vi "saveTestParameters.vi"(8 "error in (no error)":errorcluster, 11 "Logger in":refnum<class "TestDataLog.lvclass">) -> (0 "error out":errorcluster, 3 "Logger out":refnum<class "TestDataLog.lvclass">)   [LabVIEW 2013, in "TestDataLog.lvclass"]
uses:
  TestDataLog.lvclass
  <userlib>/Common/Log/Log/Log.lvclass/Log.ctl
  TestDataLog.lvclass/TestDataLog.ctl
  <vilib>/Utility/file.llb/Write To Spreadsheet File (string).vi
  <userlib>/Common/Log/Log/Log.lvclass
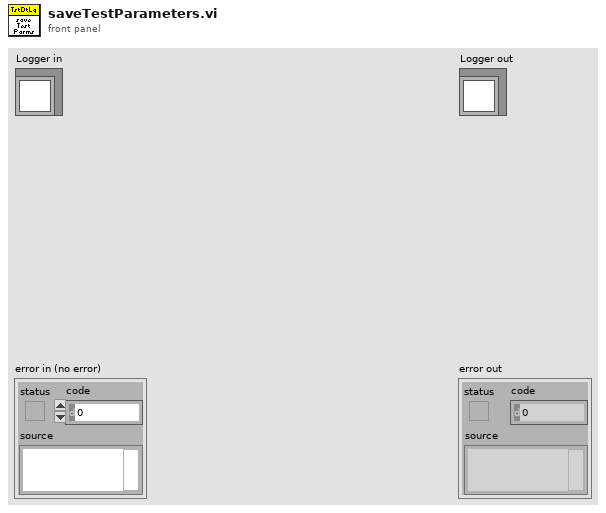
[diagram p1: front panel]
types:
  T1 = typedef "TestParameters.ctl" = cluster{"Number of cycles for complete test":u32, "Cycle profile":T2}
  T2 = typedef "CycleProfileConfig.ctl" = cluster{"Force Setpoint":dbl[unit][], "Pause After":dbl[unit][]}
  T3 = typedef "SystemController.ctl" = cluster{"PID Gains":T4, "Force Error In Range Limit":dbl[unit]}
  T4 = typedef "PIDGains.ctl" = cluster{"Proportional Gain (Kc)":dbl, "Integral Time (Ti, min)":dbl, "Derivative Time (Td, min)":dbl}
  T5 = typedef "Log.lvlib/Log.ctl" = cluster{"Log Directory":path, "Log Filename Base":string, "Max records per file":u32, "Comment":string}
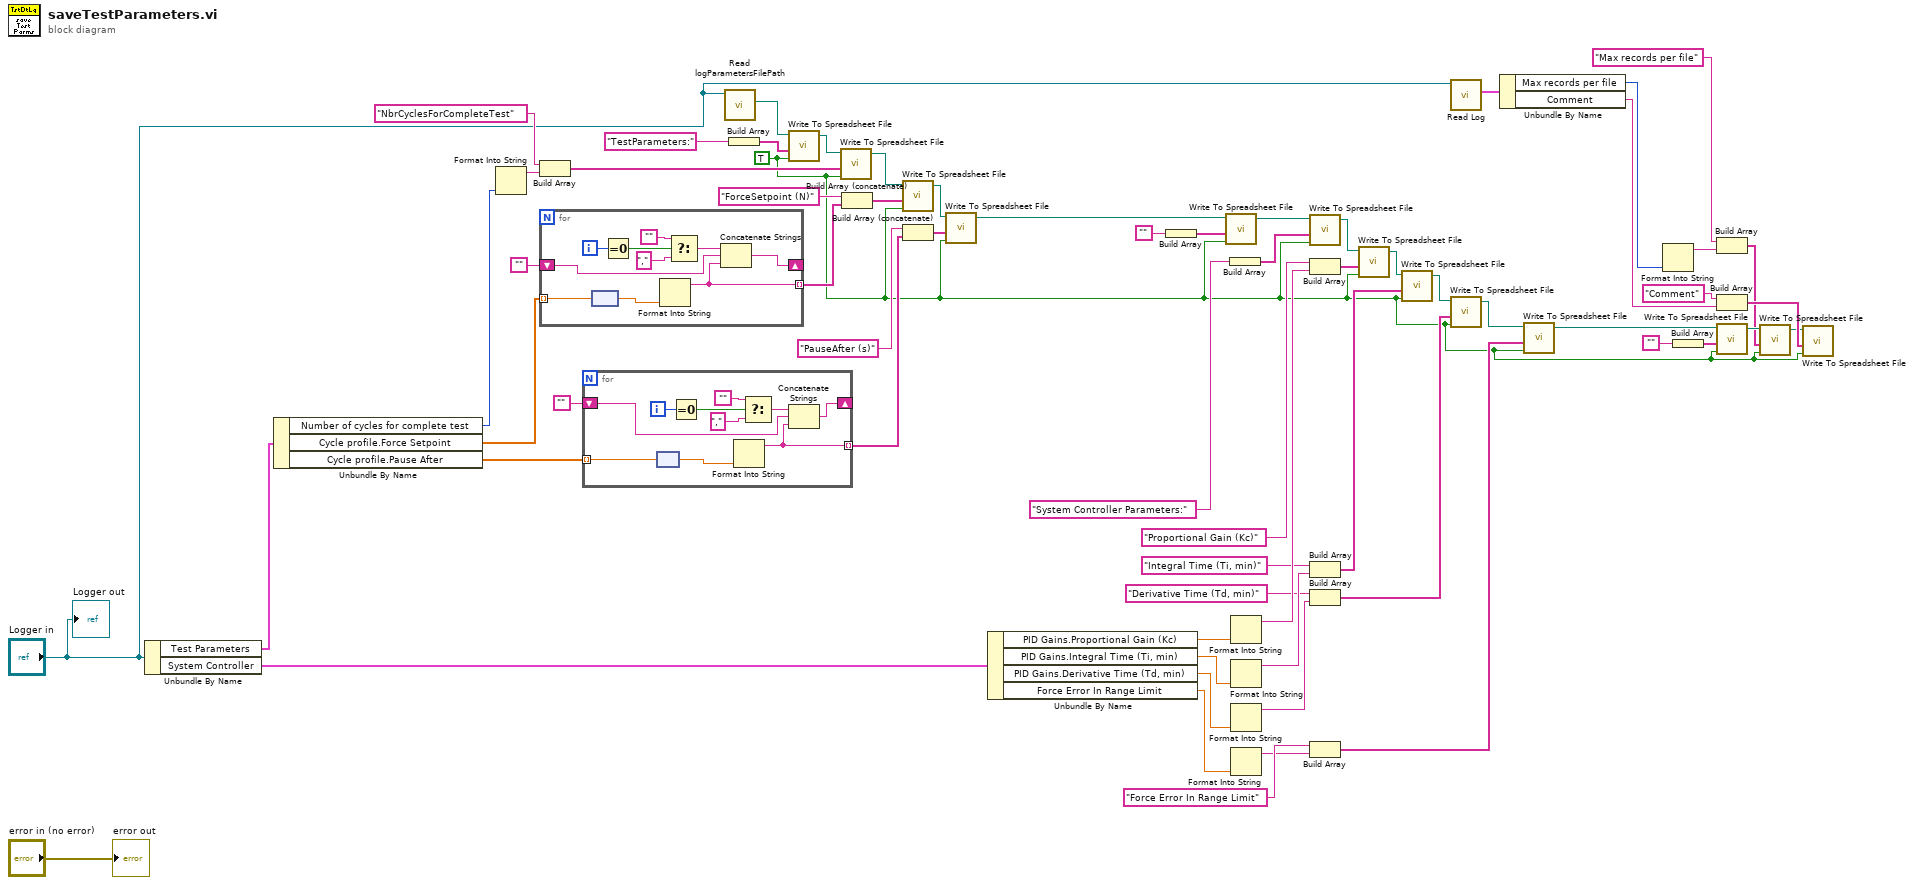
[diagram p0: block diagram]
diagram:
  w7 = TRUE ("append to file? (new file:F)")
  n1 = Unbundle By Name("Logger in") -> ("Test Parameters"=w63:T1, "System Controller"=w39:T3)
  n2 = Unbundle By Name(w63) -> ("Number of cycles for complete test"=w62:u32, "Cycle profile.Force Setpoint"=w58:dbl[unit][], "Cycle profile.Pause After"=w54:dbl[unit][])
  n3 = Format Into String(w62) -> (resulting string=w61:string)  [unwired: 3 in, 1 out]
  n4 = Build Array("NbrCyclesForCompleteTest" ("element"), w61) -> (w60:string[])
  n5 = for {
    tunnel: w58 -> [w66] mode=indexing
    shift-right: [w74] -> _
    shift-left: "" -> [w73]
    tunnel: [w67] -> w46 mode=indexing
    i -> [w72]
    n6 = node(w66) -> (w65:dbl)
    n7 = Equal To 0?(x=w72) -> (x = 0?=w71:bool)
    n8 = Format Into String(w65) -> (resulting string=w67:string)  [unwired: 3 in, 1 out]
    n9 = Select(t="", s=w71, f=",") -> (s? t:f=w68:string)
    n10 = Concatenate Strings(w68, w73, w67) -> (w74:string)
  }
  n11 = for {
    tunnel: w54 -> [w76] mode=indexing
    shift-right: [w84] -> _
    shift-left: "" -> [w83]
    tunnel: [w77] -> w45 mode=indexing
    i -> [w82]
    n12 = node(w76) -> (w75:dbl)
    n13 = Equal To 0?(x=w82) -> (x = 0?=w81:bool)
    n14 = Format Into String(w75) -> (resulting string=w77:string)  [unwired: 3 in, 1 out]
    n15 = Select(t="", s=w81, f=",") -> (s? t:f=w78:string)
    n16 = Concatenate Strings(w78, w83, w77) -> (w84:string)
  }
  n17 = call <userlib>:"Read logParametersFilePath.vi"("Logger in"="Logger in") -> ("logParametersFilePath"=w15:path)  [unwired: 9 in, 1 out]
  n18 = Build Array("TestParameters:") -> (w40:string[])
  n19 = call-poly <vilib>:"Write To Spreadsheet File.vi"("append to file? (new file:F)"=w7, "1D data"=w40, "file path (dialog if empty)"=w15) -> ("new file path (Not A Path if cancelled)"=w42:path)  [unwired: 5 in]
  n20 = call-poly <vilib>:"Write To Spreadsheet File.vi"("append to file? (new file:F)"=w7, "1D data"=w60, "file path (dialog if empty)"=w42) -> ("new file path (Not A Path if cancelled)"=w59:path)  [unwired: 5 in]
  n21 = Build Array (concatenate)("ForceSetpoint (N)" ("element"), w46) -> (w56:string[])
  n22 = call-poly <vilib>:"Write To Spreadsheet File.vi"("append to file? (new file:F)"=w7, "1D data"=w56, "file path (dialog if empty)"=w59) -> ("new file path (Not A Path if cancelled)"=w55:path)  [unwired: 5 in]
  n23 = Build Array (concatenate)("PauseAfter (s)" ("element"), w45) -> (w52:string[])
  n24 = call-poly <vilib>:"Write To Spreadsheet File.vi"("append to file? (new file:F)"=w7, "1D data"=w52, "file path (dialog if empty)"=w55) -> ("new file path (Not A Path if cancelled)"=w12:path)  [unwired: 5 in]
  n25 = Unbundle By Name(w39) -> ("PID Gains.Proportional Gain (Kc)"=w36:dbl, "PID Gains.Integral Time (Ti, min)"=w30:dbl, "PID Gains.Derivative Time (Td, min)"=w24:dbl, "Force Error In Range Limit"=w22:dbl[unit])
  n26 = Build Array("") -> (w43:string[])
  n27 = call-poly <vilib>:"Write To Spreadsheet File.vi"("append to file? (new file:F)"=w7, "1D data"=w43, "file path (dialog if empty)"=w12) -> ("new file path (Not A Path if cancelled)"=w20:path)  [unwired: 5 in]
  n28 = Build Array("System Controller Parameters:" ("element")) -> (w37:string[])
  n29 = Format Into String(w36) -> (resulting string=w34:string)  [unwired: 3 in, 1 out]
  n30 = Format Into String(w30) -> (resulting string=w29:string)  [unwired: 3 in, 1 out]
  n31 = Format Into String(w24) -> (resulting string=w23:string)  [unwired: 3 in, 1 out]
  n32 = Format Into String(w22) -> (resulting string=w21:string)  [unwired: 3 in, 1 out]
  n33 = call-poly <vilib>:"Write To Spreadsheet File.vi"("append to file? (new file:F)"=w7, "1D data"=w37, "file path (dialog if empty)"=w20) -> ("new file path (Not A Path if cancelled)"=w19:path)  [unwired: 5 in]
  n34 = Build Array("Proportional Gain (Kc)" ("element"), w34) -> (w33:string[])
  n35 = Build Array("Integral Time (Ti, min)" ("element"), w29) -> (w31:string[])
  n36 = Build Array("Derivative Time (Td, min)" ("element"), w23) -> (w26:string[])
  n37 = Build Array("Force Error In Range Limit" ("element"), w21) -> (w25:string[])
  n38 = call-poly <vilib>:"Write To Spreadsheet File.vi"("append to file? (new file:F)"=w7, "1D data"=w33, "file path (dialog if empty)"=w19) -> ("new file path (Not A Path if cancelled)"=w18:path)  [unwired: 5 in]
  n39 = call-poly <vilib>:"Write To Spreadsheet File.vi"("append to file? (new file:F)"=w7, "1D data"=w31, "file path (dialog if empty)"=w18) -> ("new file path (Not A Path if cancelled)"=w17:path)  [unwired: 5 in]
  n40 = call <userlib>:"Read Log.vi"("Log in"="Logger in") -> ("Log"=w9:T5)  [unwired: 9 in, 1 out]
  n41 = call-poly <vilib>:"Write To Spreadsheet File.vi"("append to file? (new file:F)"=w7, "1D data"=w26, "file path (dialog if empty)"=w17) -> ("new file path (Not A Path if cancelled)"=w16:path)  [unwired: 5 in]
  n42 = Unbundle By Name(w9) -> ("Max records per file"=w4:u32, "Comment"=w8:string)
  n43 = call-poly <vilib>:"Write To Spreadsheet File.vi"("append to file? (new file:F)"=w7, "1D data"=w25, "file path (dialog if empty)"=w16) -> ("new file path (Not A Path if cancelled)"=w11:path)  [unwired: 5 in]
  n44 = Format Into String(w4) -> (resulting string=w3:string)  [unwired: 3 in, 1 out]
  n45 = Build Array("") -> (w14:string[])
  n46 = Build Array("Max records per file" ("element"), w3) -> (w2:string[])
  n47 = Build Array("Comment" ("element"), w8) -> (w51:string[])
  n48 = call-poly <vilib>:"Write To Spreadsheet File.vi"("append to file? (new file:F)"=w7, "1D data"=w14, "file path (dialog if empty)"=w11) -> ("new file path (Not A Path if cancelled)"=w6:path)  [unwired: 5 in]
  n49 = call-poly <vilib>:"Write To Spreadsheet File.vi"("append to file? (new file:F)"=w7, "1D data"=w2, "file path (dialog if empty)"=w6) -> ("new file path (Not A Path if cancelled)"=w5:path)  [unwired: 5 in]
  n50 = call-poly <vilib>:"Write To Spreadsheet File.vi"("append to file? (new file:F)"=w7, "1D data"=w51, "file path (dialog if empty)"=w5) -> ()  [unwired: 5 in, 1 out]
  "error out" <- "error in (no error)"
  "Logger out" <- "Logger in"
